vi "Find Custom Device.vi"(8 "error in":errorcluster, 10 "name":string, 11 "target in":refnum<k24>) -> (0 "error out":errorcluster, 2 "custom device":u64, 3 "target out":refnum<k24>)   [LabVIEW 2020, in "Communication Bus Template Scripting.lvlib"]
uses:
  Communication Bus Template Scripting.lvlib
  NationalInstruments.VeriStand.SystemDefinitionAPI
  Constants.vi
panel:
  in  "error message":string="The item with the specified name is not an instance of this custom device."
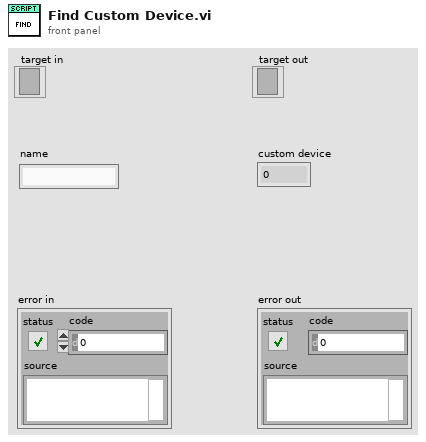
[diagram p1: front panel]
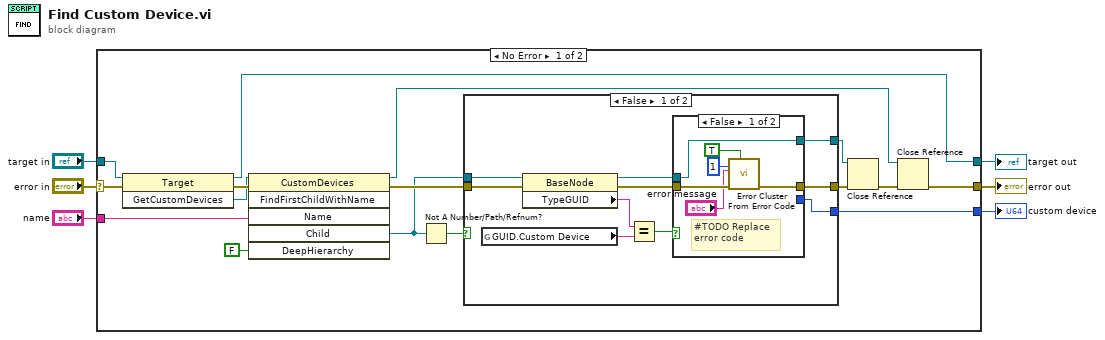
[diagram p0: block diagram]
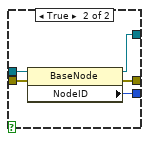
[diagram p2: hidden frame]
diagram:
  n1 = case shown="No Error" "error in" {
    selector: "error in" -> [w17 w47]
    tunnel: "target in" -> [w18 w46]
    tunnel: [w12 w47] -> w4
    tunnel: [w9 _] -> w1
    tunnel: [w14 w46] -> w3
    tunnel: "name" -> [w11 _]
    frame No Error {
      n2 = invoke on="Invoke Node" class="Target" method="GetCustomDevices"(reference=w18, error in=w17) -> (reference out=w14:refnum<k24>, error out=w22:errorcluster, "GetCustomDevices"=w21:refnum<k24>)  [unwired: 1 in]
      n3 = invoke on="Invoke Node" class="CustomDevices" method="FindFirstChildWithName"(reference=w21, error in=w22, "Name"=w11, "DeepHierarchy"=FALSE) -> (reference out=w15:refnum<k24>, error out=w13:errorcluster, "Child"=w10:refnum<k24>)  [unwired: 2 in, 3 out]
      n4 = Not A Number/Path/Refnum?(number/path/refnum=w10) -> (NaN/Path/Refnum?=w8:bool)
      n5 = case shown="False" w8 {
        tunnel: [w32 w44] -> w20
        tunnel: [w31 w45] -> w19
        tunnel: w13 -> [w29 w45]
        tunnel: w10 -> [w28 w44]
        tunnel: [w30 _] -> w9
        frame False {
          n6 = global read "Constants.vi" "GUID.Custom Device"() -> (w25:string)
          n7 = property on="Property Node" class="BaseNode"(reference=w28, error in=w29) -> (reference out=w23:refnum<k24>, error out=w24:errorcluster, "TypeGUID"=w26:string)
          n8 = Equal?(x=w26, y=w25) -> (x = y?=w27:bool)
          n9 = case shown="False" w27 {
            tunnel: [w34 w40] -> w31
            tunnel: w24 -> [w37 w42]
            tunnel: w23 -> [w38 w43]
            tunnel: [w38 w41] -> w32
            tunnel: [_ w39] -> w30
            frame False {
              # "#TODO Replace\nerror code"
              n10 = call <vilib>:"Error Cluster From Error Code.vi"("show call chain? (False)"=TRUE, "error in (no error)"=w37, "error message (\"\")"="error message", "error code (0)"=1) -> ("error out"=w34:errorcluster)  [unwired: 5 in]
            }
            frame True {
              n11 = property on="Property Node" class="BaseNode"(reference=w43, error in=w42) -> (reference out=w41:refnum<k24>, error out=w40:errorcluster, "NodeID"=w39:u64)
            }
          }
        }
        frame True {
        }
      }
      n12 = Close Reference(reference=w20, error in (no error)=w19) -> (error out=w16:errorcluster)
      n13 = Close Reference(reference=w15, error in (no error)=w16) -> (error out=w12:errorcluster)
    }
    frame Error {
    }
  }
  "error out" <- w4
  "target out" <- w3
  "custom device" <- w1
